vi "ramper3.vi"(9 "Target Setpoint":dbl, 11 "Rate":dbl) -> (1 "Ramping":bool, 3 "Current Setpoint":dbl)   [LabVIEW 2011]
panel:
  out "crement":dbl
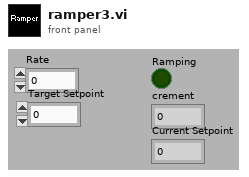
[diagram p1: front panel]
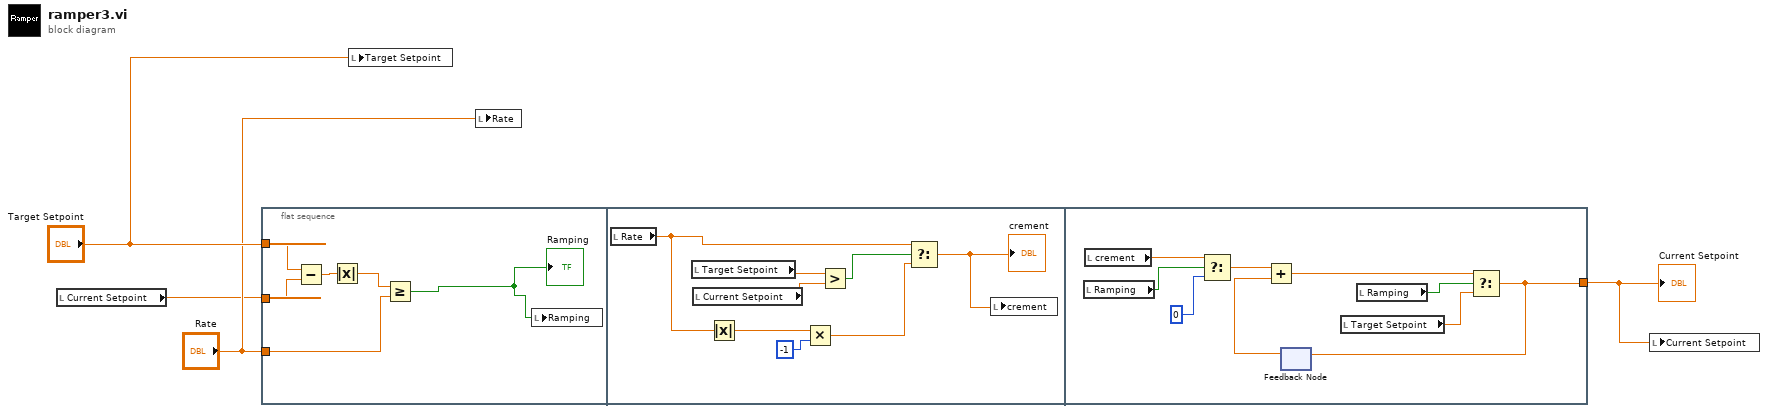
[diagram p0: block diagram]
diagram:
  n1 = local read "Current Setpoint"() -> (w1:dbl)
  n2 = flat-sequence {
    tunnel: "Target Setpoint" -> [w6]
    tunnel: w1 -> [w8]
    tunnel: "Rate" -> [w7]
    tunnel: [w20] -> w2
    frame #0 {
      n3 = Subtract(x=w6, y=w8) -> (x-y=w9:dbl)
      n4 = Absolute Value(x=w9) -> (abs(x)=w10:dbl)
      n5 = Greater Or Equal?(x=w10, y=w7) -> (x >= y?=w5:bool)
      "Ramping" <- w5
      n6 = local write "Ramping"(w5) -> ()
    }
    frame #1 {
      n7 = local read "Rate"() -> (w15:dbl)
      n8 = local read "Target Setpoint"() -> (w18:dbl)
      n9 = local read "Current Setpoint"() -> (w17:dbl)
      n10 = Absolute Value(x=w15) -> (abs(x)=w14:dbl)
      n11 = Multiply(x=w14, y=-1) -> (x*y=w12:dbl)
      n12 = Greater?(x=w18, y=w17) -> (0:w16:bool)
      n13 = Select(t=w15, s=w16, f=w12) -> (s? t:f=w11:dbl)
      "crement" <- w11
      n14 = local write "crement"(w11) -> ()
    }
    frame #2 {
      n15 = local read "Ramping"() -> (w26:bool)
      n16 = local read "crement"() -> (w27:dbl)
      n17 = Select(t=w27, s=w26, f=0) -> (s? t:f=w24:dbl)
      n18 = feedback #1() -> (w21:dbl)  [unwired: 1 out]
      n19 = Add(x=w24, y=w21) -> (x+y=w23:dbl)
      n20 = local read "Target Setpoint"() -> (w22:dbl)
      n21 = local read "Ramping"() -> (w19:bool)
      n22 = Select(t=w23, s=w19, f=w22) -> (s? t:f=w20:dbl)
      n23 = feedback-in #1(w20) -> ()
    }
  }
  n24 = local write "Target Setpoint"("Target Setpoint") -> ()
  n25 = local write "Rate"("Rate") -> ()
  n26 = local write "Current Setpoint"(w2) -> ()
  "Current Setpoint" <- w2
